vi "LED+Intensity[1] final.vi"() -> ()   [LabVIEW 2022 SP3]
panel:
  in  "stop":bool
  in  "milliseconds to wait 4":u32
  in  "write buffer 5":string
  in  "milliseconds to wait 3":u32
  in  "write buffer 4":string
  in  "milliseconds to wait 2":u32
  in  "milliseconds to wait":u32
  in  "write buffer 3":string
  in  "write buffer 2":string
  in  "write buffer":string
  in  "VISA resource name":refnum<visa-resource-name>
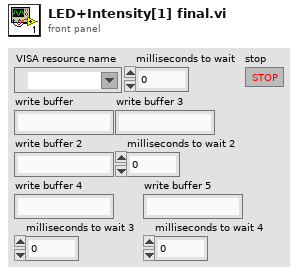
[diagram p1: front panel]
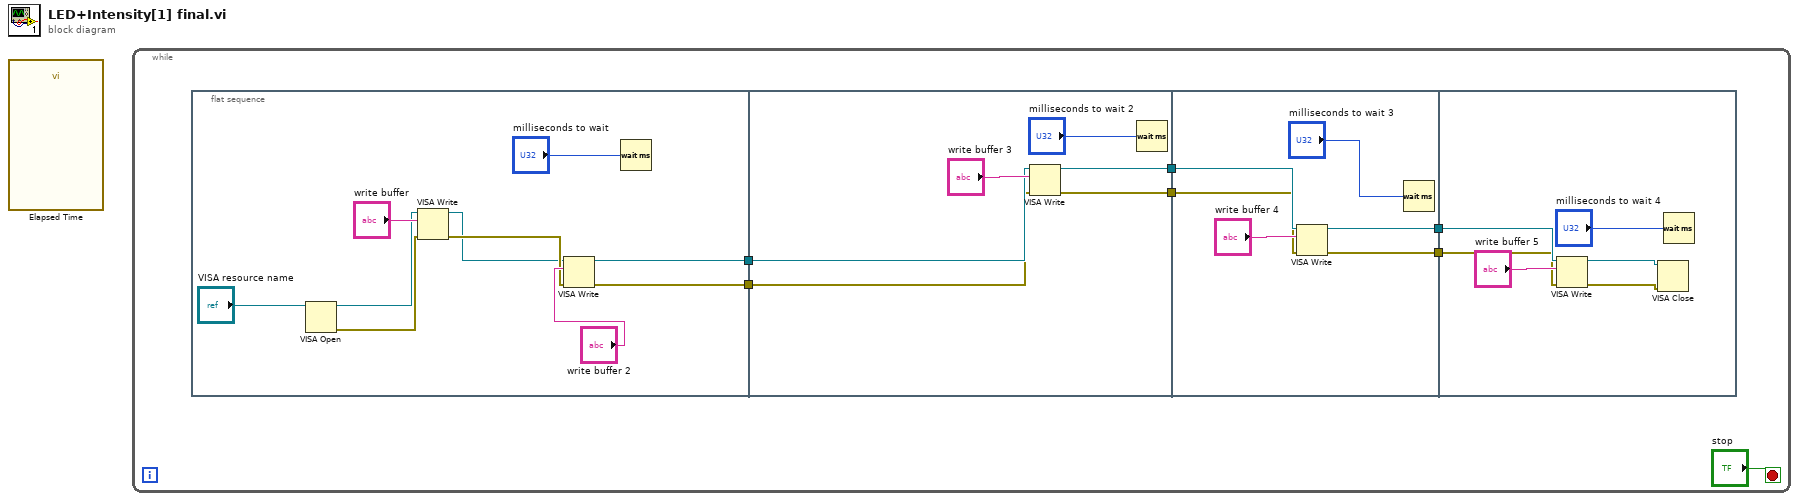
[diagram p0: block diagram]
diagram:
  n1 = call "Elapsed Time"() -> ()  [unwired: 12 in, 8 out]
  n2 = while {
    stop <- "stop" stop-if-true
    n3 = flat-sequence {
      tunnel: [w10] -> w7
      tunnel: [w9] -> w6
      tunnel: w7 -> [w22]
      tunnel: w6 -> [w21]
      tunnel: [w19] -> w5
      tunnel: [w18] -> w4
      tunnel: w5 -> [w27]
      tunnel: w4 -> [w26]
      tunnel: [w25] -> w3
      tunnel: [w24] -> w2
      tunnel: w3 -> [w33]
      tunnel: w2 -> [w32]
      frame #0 {
        n4 = VISA Open(VISA resource name="VISA resource name") -> (VISA resource name=w12:refnum<visa-resource-name>, error out=w15:errorcluster)  [unwired: 4 in]
        n5 = VISA Write(VISA resource name=w12, write buffer="write buffer", error in (no error)=w15) -> (VISA resource name out=w14:refnum<visa-resource-name>, error out=w16:errorcluster)  [unwired: 1 out]
        n6 = VISA Write(VISA resource name=w14, write buffer="write buffer 2", error in (no error)=w16) -> (VISA resource name out=w10:refnum<visa-resource-name>, error out=w9:errorcluster)  [unwired: 1 out]
        n7 = Wait (ms)(milliseconds to wait="milliseconds to wait") -> ()  [unwired: 1 out]
      }
      frame #1 {
        n8 = VISA Write(VISA resource name=w22, write buffer="write buffer 3", error in (no error)=w21) -> (VISA resource name out=w19:refnum<visa-resource-name>, error out=w18:errorcluster)  [unwired: 1 out]
        n9 = Wait (ms)(milliseconds to wait="milliseconds to wait 2") -> ()  [unwired: 1 out]
      }
      frame #2 {
        n10 = VISA Write(VISA resource name=w27, write buffer="write buffer 4", error in (no error)=w26) -> (VISA resource name out=w25:refnum<visa-resource-name>, error out=w24:errorcluster)  [unwired: 1 out]
        n11 = Wait (ms)(milliseconds to wait="milliseconds to wait 3") -> ()  [unwired: 1 out]
      }
      frame #3 {
        n12 = VISA Write(VISA resource name=w33, write buffer="write buffer 5", error in (no error)=w32) -> (VISA resource name out=w31:refnum<visa-resource-name>, error out=w30:errorcluster)  [unwired: 1 out]
        n13 = VISA Close(VISA resource name=w31, error in (no error)=w30) -> ()  [unwired: 1 out]
        n14 = Wait (ms)(milliseconds to wait="milliseconds to wait 4") -> ()  [unwired: 1 out]
      }
    }
  }
